vi "Generate U Rotation Matrix.vi"(8 "error in (no error)":errorcluster, 10 "SLAM In":T2) -> (0 "error out":errorcluster, 2 "SLAM Out":T2, 3 "Rotation matrix":T1)   [LabVIEW 2009]
uses:
  Controls/SLAM.ctl
  <vilib>/Analysis/Matrix/Datatypes/RealMatrix.ctl
  <vilib>/Analysis/Matrix/NI_Matrix.lvlib
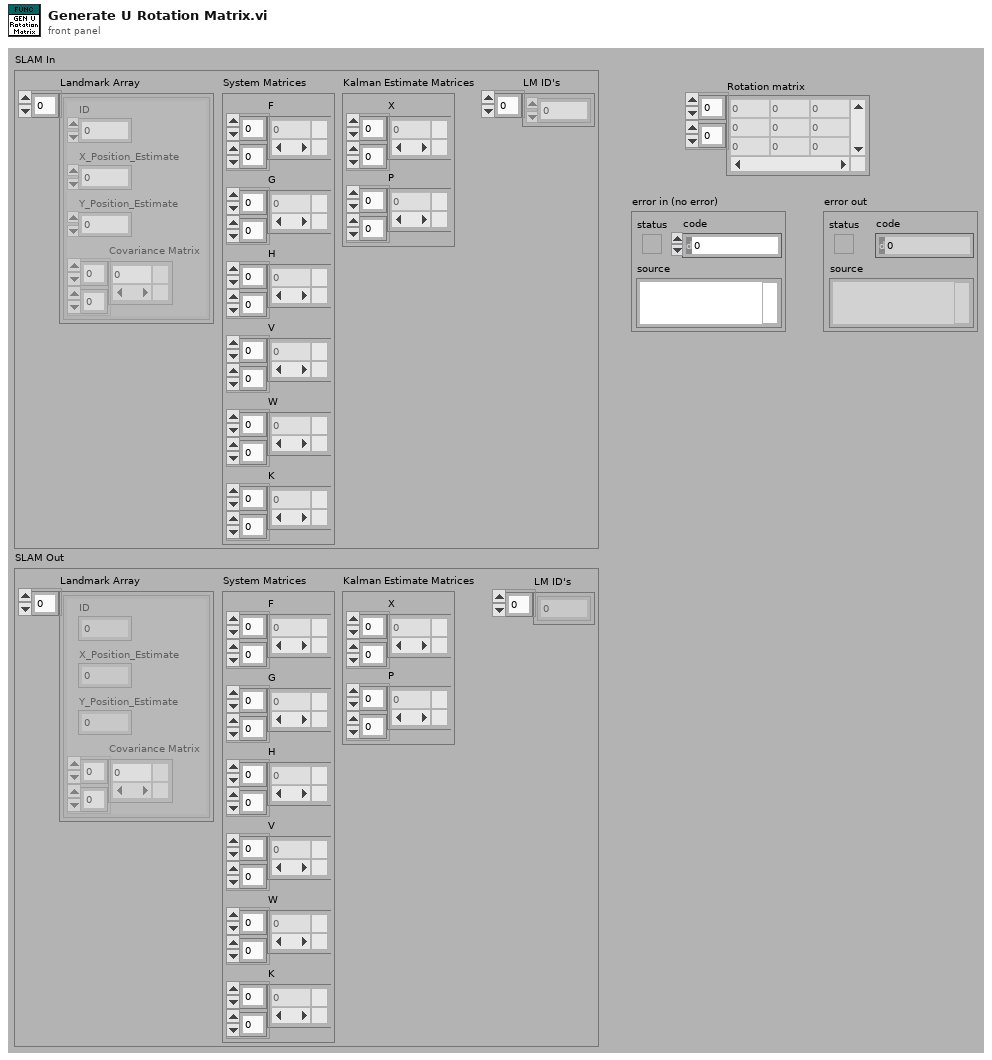
[diagram p1: front panel]
types:
  T1 = typedef "NI_Matrix.lvlib/RealMatrix.ctl" = dbl[][]
  T2 = typedef "SLAM.ctl" = cluster{"Landmark Array":cluster{"ID":dbl, "X_Position_Estimate":dbl, "Y_Position_Estimate":dbl, "Covariance Matrix":T1}[], "System Matrices":cluster{"F":T1, "G":T1, "H":T1, "V":T1, "W":T1, "K":T1}, "Kalman Estimate Matrices":cluster{"X":T1, "P":T1}, "LM ID's":dbl[]}
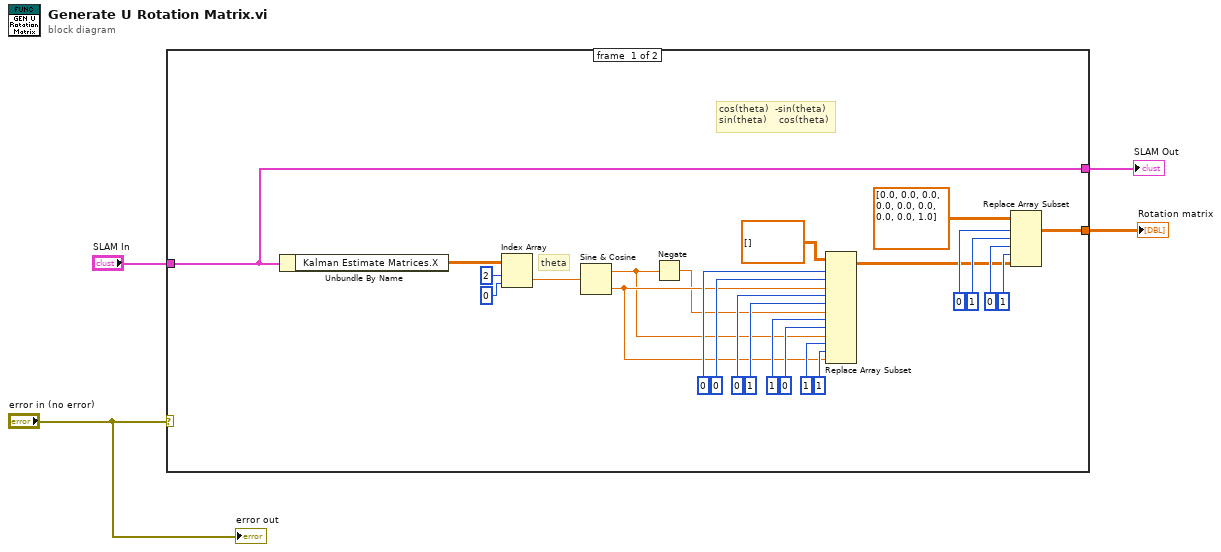
[diagram p0: block diagram]
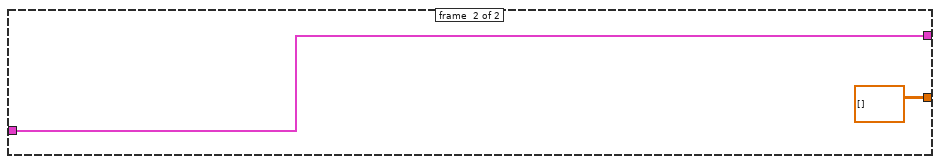
[diagram p2: hidden frame]
diagram:
  n1 = case shown="No Error" "error in (no error)" {
    tunnel: "SLAM In" -> [w12 w30]
    tunnel: [w12 w30] -> w2
    tunnel: [w5 T1 [] ("Real Matrix")] -> w1
    frame #0 {
      # "cos(theta)  -sin(theta)\nsin(theta)    cos(theta)"
      # "theta"
      n2 = Unbundle By Name(w12) -> ("Kalman Estimate Matrices.X"=w17:T1)
      n3 = Index Array(array=w17, index (row)=2, index (col)=0) -> (element=w26:dbl)
      n4 = Sine & Cosine(0:w26) -> (1:w15:dbl, 2:w16:dbl)
      n5 = Negate(x=w15) -> (-x=w14:dbl)
      n6 = Replace Array Subset(array=T1 [] ("matrix"), new element #1=w16, index (row) #1=0 ("disabled index (row)"), index (col) #1=0 ("disabled index (row)"), new element #2=w14, index (row) #2=0 ("disabled index (row)"), index (col) #2=1 ("disabled index (row)"), new element #3=w15, index (row) #3=1 ("disabled index (row)"), index (col) #3=0 ("disabled index (row)"), new element #4=w16, index (row) #4=1 ("disabled index (row)"), index (col) #4=1 ("disabled index (row)")) -> (w6:T1)
      n7 = Replace Array Subset(array=T1 [[0.0, 0.0, 0.0], [0.0, 0.0, 0.0], [0.0, 0.0, 1.0]] ("matrix"), new element=w6, index (dim 0)=0 ("row 1"), index (dim 1)=1 ("row 1"), index (dim 2)=0 ("row 1"), index (dim 3)=1 ("row 1")) -> (w5:T1)
    }
    frame #1 {
    }
  }
  "SLAM Out" <- w2
  "Rotation matrix" <- w1
  "error out" <- "error in (no error)"
